vi "TrapezoidMotionProfie.vi"(6 "Start Time":dbl, 7 "Constraints":T2, 8 "Final Velocity":dbl, 9 "Initial Velocity":dbl, 10 "Theta":dbl[](array[numeric]), 11 "Arc Length":dbl[](array[numeric])) -> (2 "Final Time":dbl, 3 "Motion Cluster":T1(array[cluster]))   [LabVIEW 2016]
panel:
  out "XY Graph":cluster{dbl, "Initial Velocity":dbl}[](graph)
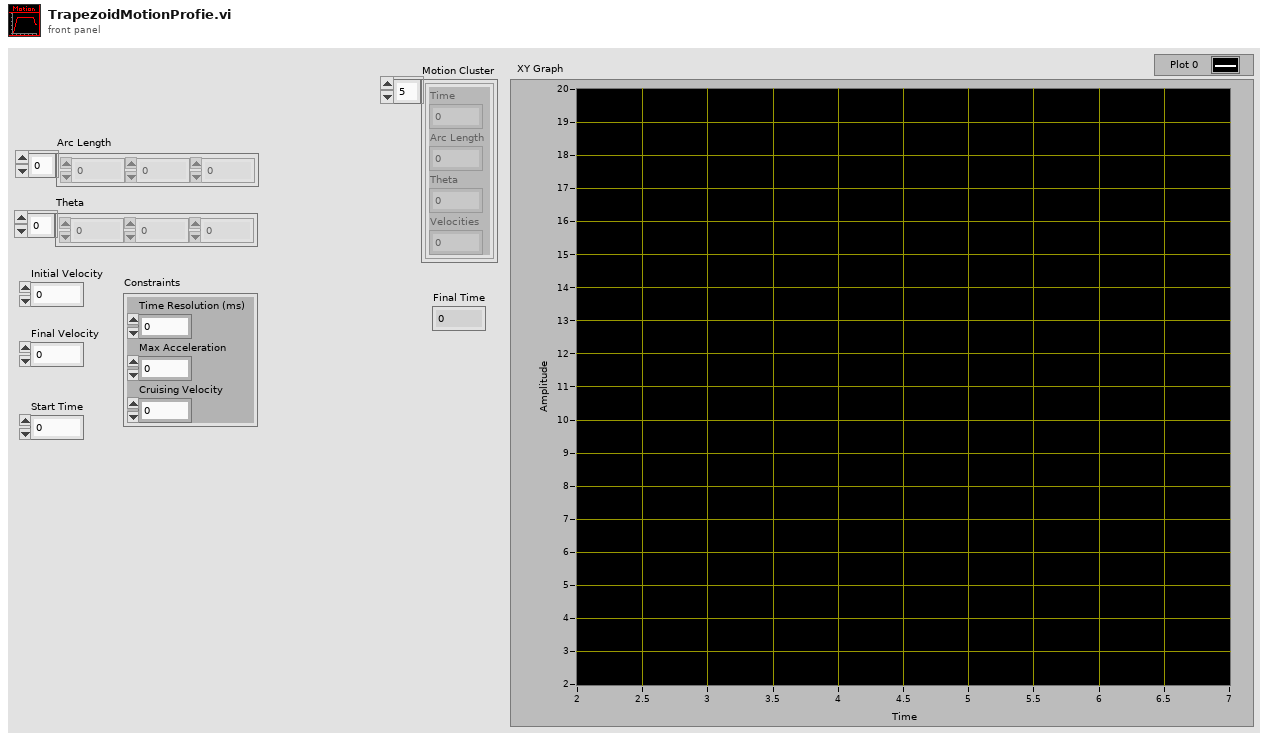
[diagram p1: front panel]
types:
  T1 = cluster{"Time":dbl, "Arc Length":dbl, "Theta":dbl, "Velocities":dbl}[]
  T2 = cluster{"Time Resolution (ms)":i32, "Max Acceleration":dbl, "Cruising Velocity":dbl}
  T3 = cluster{dbl, "Initial Velocity":dbl, "Initial Velocity":dbl, "Initial Velocity":dbl}[]
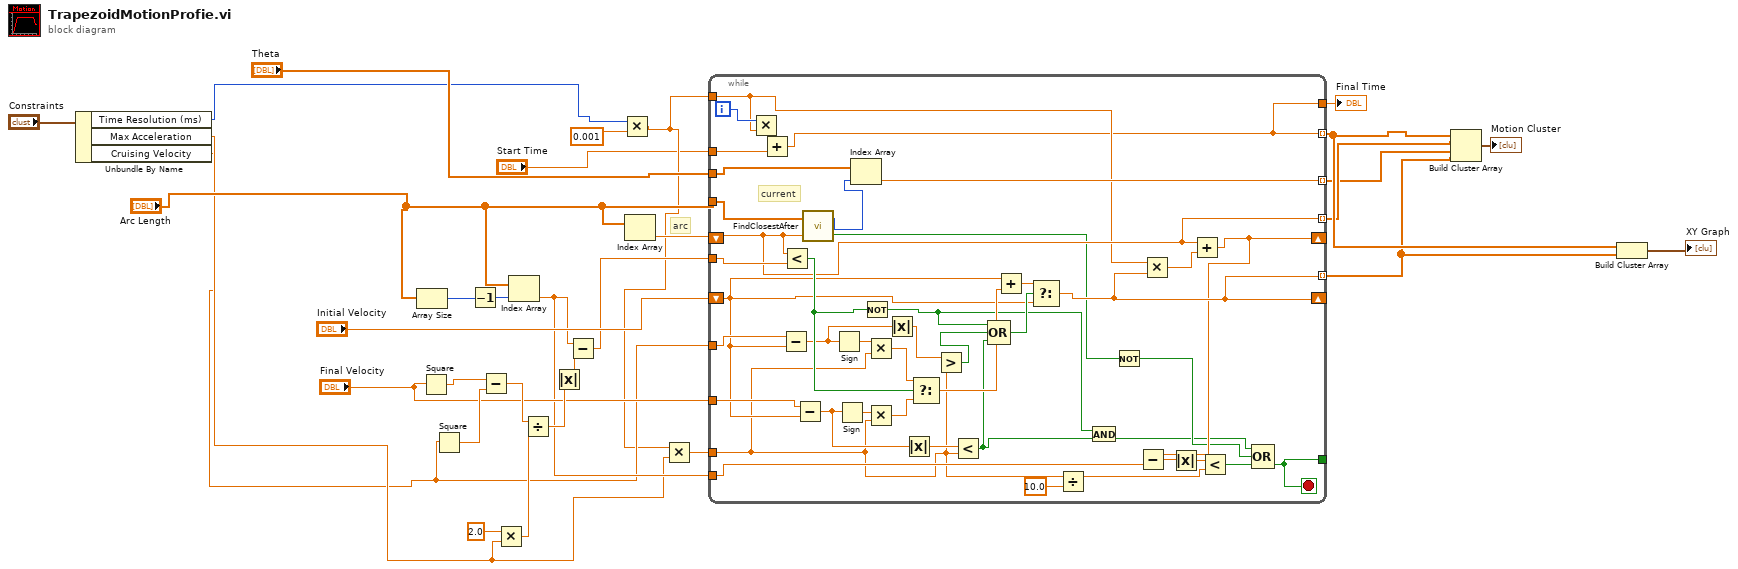
[diagram p0: block diagram]
diagram:
  # "arc"
  n1 = Unbundle By Name("Constraints") -> ("Time Resolution (ms)"=w10:i32, "Max Acceleration"=w12:dbl, "Cruising Velocity"=w11:dbl)
  n2 = Array Size(array="Arc Length") -> (size(s)=w31:i32)
  n3 = Square(x="Final Velocity") -> (x^2=w27:dbl)
  n4 = Square(x=w11) -> (x^2=w28:dbl)
  n5 = Decrement(x=w31) -> (x-1=w30:i32)
  n6 = Subtract(x=w27, y=w28) -> (x-y=w26:dbl)
  n7 = Multiply(x=2.0, y=w12) -> (x*y=w24:dbl)
  n8 = Index Array(array="Arc Length", index=w30) -> (element=w16:dbl)
  n9 = Divide(x=w26, y=w24) -> (x/y=w23:dbl)
  n10 = Absolute Value(x=w23) -> (abs(x)=w17:dbl)
  n11 = Subtract(x=w16, y=w17) -> (x-y=w22:dbl)
  n12 = Multiply(x=w10, y=0.001 ("Start Time")) -> (x*y=w3:dbl)
  n13 = Index Array(array="Arc Length") -> (element=w21:dbl)  [unwired: 1 in]
  n14 = Multiply(x=w3, y=w12) -> (x*y=w20:dbl)
  n15 = while {
    tunnel: [w40] -> w8 mode=indexing
    tunnel: w11 -> [w64]
    shift-right: [w54] -> _
    shift-left: "Initial Velocity" -> [w56]
    tunnel: "Arc Length" -> [w47]
    tunnel: "Theta" -> [w73]
    tunnel: w22 -> [w71]
    shift-right: [w52] -> _
    shift-left: w21 -> [w53]
    tunnel: [w72] -> w6 mode=indexing
    tunnel: w20 -> [w35]
    tunnel: "Final Velocity" -> [w69]
    tunnel: [w53] -> w7 mode=indexing
    tunnel: [w54] -> w5 mode=indexing
    tunnel: w16 -> [w51]
    tunnel: [w46] -> _
    tunnel: w3 -> [w41]
    tunnel: "Start Time" -> [w42]
    tunnel: [w40] -> w1
    i -> [w74]
    stop <- w46 stop-if-true
    # "current"
    n16 = Multiply(x=w74, y=w41) -> (x*y=w43:dbl)
    n17 = Add(x=w43, y=w42) -> (x+y=w40:dbl)
    n18 = Subtract(x=w64, y=w56) -> (x-y=w60:dbl)
    n19 = Less?(x=w53, y=w71) -> (x < y?=w63:bool)
    n20 = Subtract(x=w69, y=w56) -> (x-y=w37:dbl)
    n21 = call "FindClosestAfter.vi"("Setpoint"=w53, "Sorted Array"=w47) -> ("Valid?"=w45:bool, "Index next to setpoint"=w70:i32)
    n22 = Sign(1:w60) -> (0:w68:dbl)
    n23 = Sign(1:w37) -> (0:w67:dbl)
    n24 = Index Array(array=w73, index=w70) -> (element=w72:dbl)
    n25 = Not(x=w63) -> (.not. x?=w32:bool)
    n26 = Multiply(x=w68, y=w35) -> (x*y=w65:dbl)
    n27 = Multiply(x=w67, y=w35) -> (x*y=w66:dbl)
    n28 = Absolute Value(x=w60) -> (abs(x)=w59:dbl)
    n29 = Absolute Value(x=w37) -> (abs(x)=w36:dbl)
    n30 = Select(t=w65, s=w63, f=w66) -> (s? t:f=w58:dbl)
    n31 = Greater?(x=w59, y=w35) -> (0:w61:bool)
    n32 = Less?(x=w36, y=w35) -> (x < y?=w34:bool)
    n33 = Compound Arithmetic op=OR(w32, w61, w34) -> (w62:bool)
    n34 = Add(x=w56, y=w58) -> (x+y=w57:dbl)
    n35 = Select(t=w57, s=w62, f=w56) -> (s? t:f=w54:dbl)
    n36 = Divide(x=w35, y=10.0) -> (x/y=w39:dbl)
    n37 = And(x=w32, y=w34) -> (x .and. y?=w33:bool)
    n38 = Not(x=w45) -> (.not. x?=w44:bool)
    n39 = Multiply(x=w41, y=w54) -> (x*y=w55:dbl)
    n40 = Add(x=w53, y=w55) -> (x+y=w52:dbl)
    n41 = Subtract(x=w52, y=w51) -> (x-y=w50:dbl)
    n42 = Absolute Value(x=w50) -> (abs(x)=w49:dbl)
    n43 = Less?(x=w49, y=w39) -> (x < y?=w48:bool)
    n44 = Compound Arithmetic op=OR(w33, w44, w48) -> (w46:bool)
  }
  "Final Time" <- w1
  n45 = Build Cluster Array(w8, w7, w6, w5) -> (→"Motion Cluster":T3)
  n46 = Build Cluster Array(w8, w5) -> (→"XY Graph":cluster{dbl, "Initial Velocity":dbl}[])
